vi "output.vi"(8 "error in (no error)":errorcluster, 10 "Output [on/off]":bool, 11 "PSP-603 in":refnum<class "PSP-603.lvclass">) -> (0 "error out":errorcluster, 3 "PSP-603 out":refnum<class "PSP-603.lvclass">)   [LabVIEW 2025, in "Power Supply.lvlib" / "PSP-603.lvclass"]
uses:
  PSP-603.lvclass
  PSP-603.lvclass/PSP-603.ctl
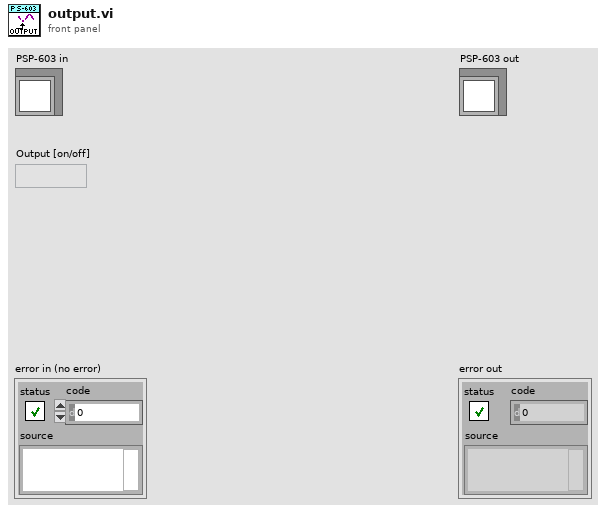
[diagram p1: front panel]
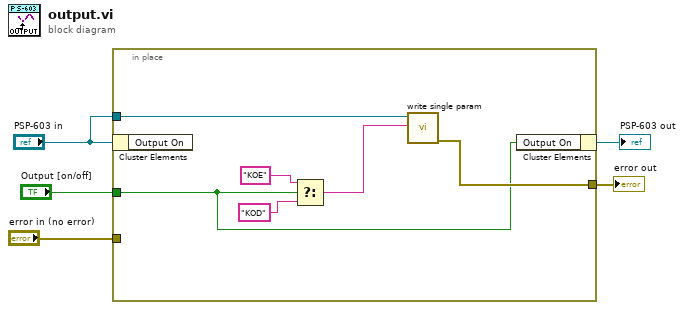
[diagram p0: block diagram]
diagram:
  n1 = in-place {
    in-place-border: "Output [on/off]" -> [w9]
    in-place-border: "PSP-603 in" -> [w11]
    in-place-border: [w10] -> w2
    in-place-border: "error in (no error)" -> [_]
    n2 = in-place-cluster #1("PSP-603 in") -> ()  [unwired: 1 out]
    n3 = Select(t="KOE" ("string"), s=w9, f="KOD" ("string")) -> (s? t:f=w6:string)
    n4 = call-dynamic "write single param.vi"("string"=w6, "PSP-603 in"=w11) -> ("error out"=w10:errorcluster)  [unwired: 8 in, 1 out]
    n5 = in-place-cluster #1("Output On"=w9) -> (→"PSP-603 out":refnum<class "PSP-603.lvclass">)
  }
  "error out" <- w2
